vi "get Request Channel.vi"(8 "error in (no error)":errorcluster, 11 "Actor API in":refnum<class "Actor API.lvclass">) -> (0 "error out":errorcluster, 2 "Request Channel":refnum<class "Messenger.lvclass">, 3 "Actor API out":refnum<class "Actor API.lvclass">)   [LabVIEW 2015, in "Actor API.lvclass"]
uses:
  Actor API.lvclass
  Messaging/Messenger/Messenger.lvclass
  Actor API.lvclass/Actor API.ctl
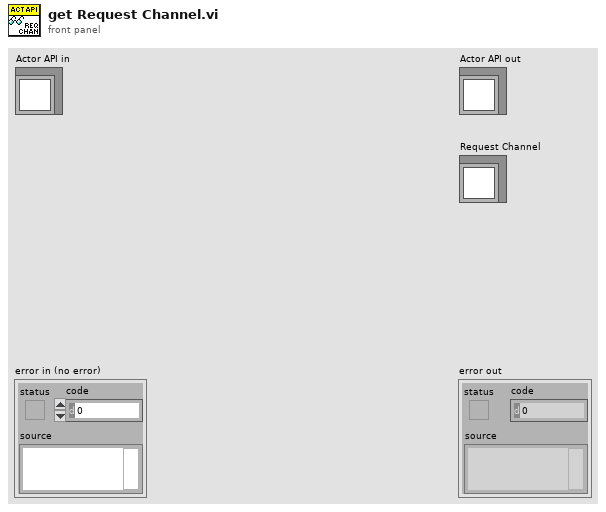
[diagram p1: front panel]
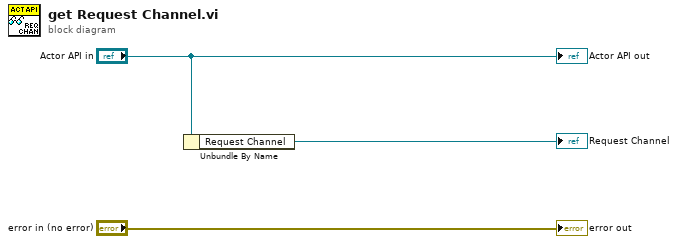
[diagram p0: block diagram]
diagram:
  n1 = Unbundle By Name("Actor API in") -> ("Request Channel"=→"Request Channel":refnum<class "Messenger.lvclass">)
  "error out" <- "error in (no error)"
  "Actor API out" <- "Actor API in"
